vi "connecting to found devices.vi"(8 "error in (no error)":errorcluster, 11 "Thorcam in":refnum<class "Thorcam.lvclass">) -> (0 "error out":errorcluster, 2 "Number of Cameras":i32, 3 "Thorcam out":refnum<class "Thorcam.lvclass">)   [LabVIEW 2012, in "Thorcam.lvclass"]
uses:
  Thorcam.lvclass
  Thorcam.lvclass/Thorcam.ctl
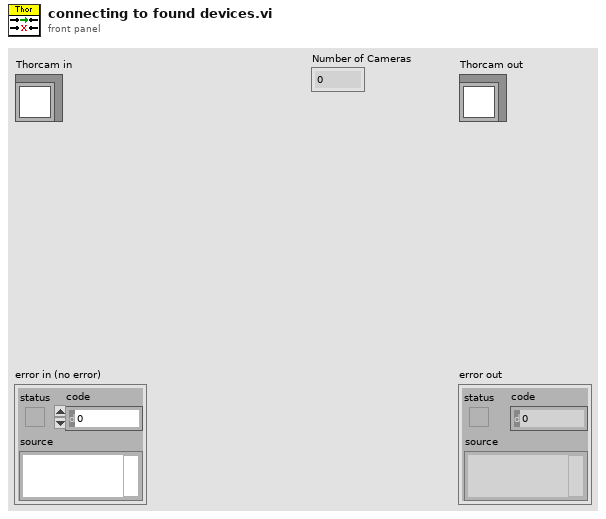
[diagram p1: front panel]
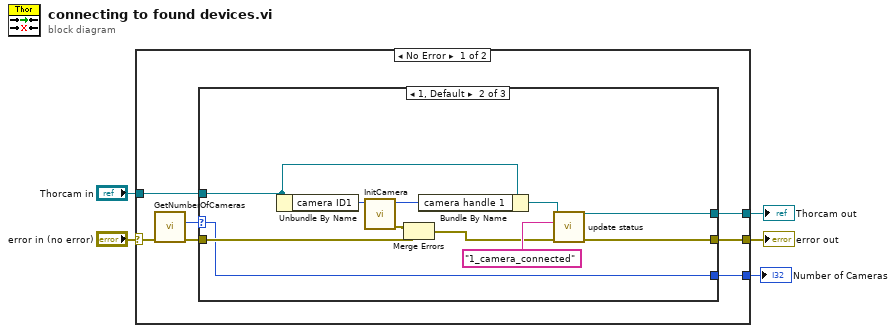
[diagram p0: block diagram]
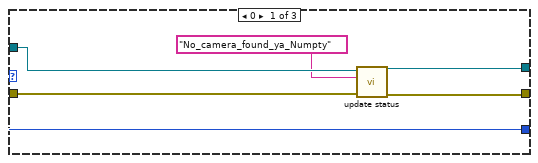
[diagram p2: hidden frame]
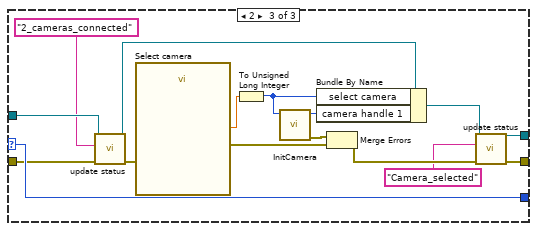
[diagram p3: hidden frame]
diagram:
  n1 = case shown="No Error" "error in (no error)" {
    selector: "error in (no error)" -> [w12 w47]
    tunnel: [w10 w47] -> w4
    tunnel: [w7 w46] -> w2
    tunnel: "Thorcam in" -> [w8 w46]
    tunnel: [w6 _] -> w1
    frame No Error {
      n2 = call <instrlib>:"GetNumberOfCameras.vi"("error in"=w12) -> ("error out"=w11:errorcluster, "Number of Cameras"=w9:i32)  [unwired: 9 in]
      n3 = case shown="1, Default" w9 {
        selector: w9 -> [w13 w22 w38]
        tunnel: [w17 w25 w43] -> w10
        tunnel: w11 -> [w18 w28 w34]
        tunnel: w8 -> [w16 w20 w32]
        tunnel: [w15 w24 w40] -> w7
        tunnel: [w13 w22 w38] -> w6
        frame 0 {
          n4 = call-dynamic "update status.vi"("error in (no error)"=w18, "status in"="No_camera_found_ya_Numpty", "Thorcam in"=w16) -> ("error out"=w17:errorcluster, "Thorcam out"=w15:refnum<class "Thorcam.lvclass">)  [unwired: 7 in]
        }
        frame 1, Default {
          n5 = Unbundle By Name(w20) -> ("camera ID1"=w21:u32)
          n6 = call <instrlib>:"InitCamera.vi"("Camera ID"=w21) -> ("error out"=w29:errorcluster, "Camera Handle Out"=w23:u32)  [unwired: 9 in]
          n7 = Merge Errors(w29, w28) -> (w26:errorcluster)
          n8 = Bundle By Name(cluster=w20, "camera handle 1"=w23) -> (w19:refnum<class "Thorcam.lvclass">)
          n9 = call-dynamic "update status.vi"("error in (no error)"=w26, "status in"="1_camera_connected" ("String In"), "Thorcam in"=w19) -> ("error out"=w25:errorcluster, "Thorcam out"=w24:refnum<class "Thorcam.lvclass">)  [unwired: 7 in]
        }
        frame 2 {
          n10 = call-dynamic "update status.vi"("error in (no error)"=w34, "status in"="2_cameras_connected", "Thorcam in"=w32) -> ("error out"=w33:errorcluster, "Thorcam out"=w31:refnum<class "Thorcam.lvclass">)  [unwired: 7 in]
          n11 = call "Select camera"("error in (no error)"=w33) -> ("Camera"=w36:dbl, "error out"=w37:errorcluster)  [unwired: 16 in, 1 out]
          n12 = To Unsigned Long Integer(number=w36) -> (unsigned 32bit integer=w35:u32)
          n13 = call <instrlib>:"InitCamera.vi"("Camera ID"=w35) -> ("error out"=w45:errorcluster, "Camera Handle Out"=w44:u32)  [unwired: 9 in]
          n14 = Bundle By Name(cluster=w31, "select camera"=w35, "camera handle 1"=w44) -> (w41:refnum<class "Thorcam.lvclass">)
          n15 = Merge Errors(w45, w37) -> (w42:errorcluster)
          n16 = call-dynamic "update status.vi"("error in (no error)"=w42, "status in"="Camera_selected", "Thorcam in"=w41) -> ("error out"=w43:errorcluster, "Thorcam out"=w40:refnum<class "Thorcam.lvclass">)  [unwired: 7 in]
        }
      }
    }
    frame Error {
    }
  }
  "error out" <- w4
  "Thorcam out" <- w2
  "Number of Cameras" <- w1
